vi "Main.vi"(11 "Module Admin":refnum<class "Delacor_lib_QMH_Cloneable Module Admin.lvclass">) -> ()   [LabVIEW 2025, in "Torque Transducer.lvlib"]
doc: "This template is based off of the Queued Message Handler design pattern and the Queued Message Handler project template that ships with LabVIEW.\n\nThe main difference is that the queue is private to this module and communication between modules is performed via Broadcast and Request events.\n\nRequest events are wrapped in public API methods and are handled in the Event Handling Loop (EHL) of this VI. Any module can register for Broadcast events sent by this module. The EHL generates messages based on user interface actions.\n\nThe Message Handling Loop (MHL) processes messages generated by the EHL, or by other messages. The messages are string values, so new messages can be added easily to the Message Cases case structure in the MHL. Each message cluster can also provide an optional value for Message Data, which is a variant that can be converted to whatever message-specific data is required.\n_____\nBased on DQMH Dev Tools: Project Template 7.1.2.1547."
uses:
  Torque Transducer.lvlib
  <vilib>/Delacor/Delacor QMH/Libraries/Cloneable Module Admin_class/Delacor_lib_QMH_Cloneable Module Admin.lvclass
  Module Data--cluster.ctl
  Classes/Torque Transducer/Torque Transducer.lvclass
  <vilib>/Delacor/Delacor QMH/Libraries/Cloneable Module Admin_class/Delacor_lib_QMH_Cloneable Module Admin.lvclass/Delacor_lib_QMH_Cloneable Module Admin.ctl
  <vilib>/Delacor/Delacor QMH/Libraries/Message Queue_class/Delacor_lib_QMH_Message Queue.lvclass/Delacor_lib_QMH_Message Queue.ctl
  Stop Argument--cluster.ctl
  <vilib>/Delacor/Delacor QMH/Libraries/Module Admin_class/Delacor_lib_QMH_Module Admin.lvclass/Delacor_lib_QMH_Module Admin.ctl
  Get Torque DVR Argument--cluster.ctl
  Get Torque DVR (Reply Payload)--cluster.ctl
  read torque Argument--cluster.ctl
  read torque (Reply Payload)--cluster.ctl
  close Argument--cluster.ctl
  close (Reply Payload)--cluster.ctl
  read config Argument--cluster.ctl
  read config (Reply Payload)--cluster.ctl
  init daq Argument--cluster.ctl
  init daq (Reply Payload)--cluster.ctl
  <vilib>/Utility/miscctls.llb/LVPointTypeDef.ctl
  <vilib>/Delacor/Delacor QMH/Libraries/Cloneable Module Admin_class/Delacor_lib_QMH_Get Module ID.vi
  <vilib>/Delacor/Delacor QMH/Libraries/Message Queue_class/Delacor_lib_QMH_Enqueue Message (Single).vi
  <vilib>/Delacor/Delacor QMH/Libraries/Module Admin_class/Delacor_lib_QMH_Get External Launch.vi
  <vilib>/Delacor/Delacor QMH/Libraries/Message Queue_class/Delacor_lib_QMH_Message Queue.lvclass
panel:
  out "Stop the VI":bool
  out "error out":errorcluster
  out "Status":string
  in  "Simulate EHL Error":bool
  in  "Simulate MHL Error":bool
  # "Other processes communicate with this Module via its Public API (wrappers for its Request Events).\n\nThis Module communicates with other processes via its Broadcast Events.\nAny process that wants to receive these messages can register for this module's Broadcast events."
  # "This template is for the DQMH framework. See the block diagram for more information on how to use this template."
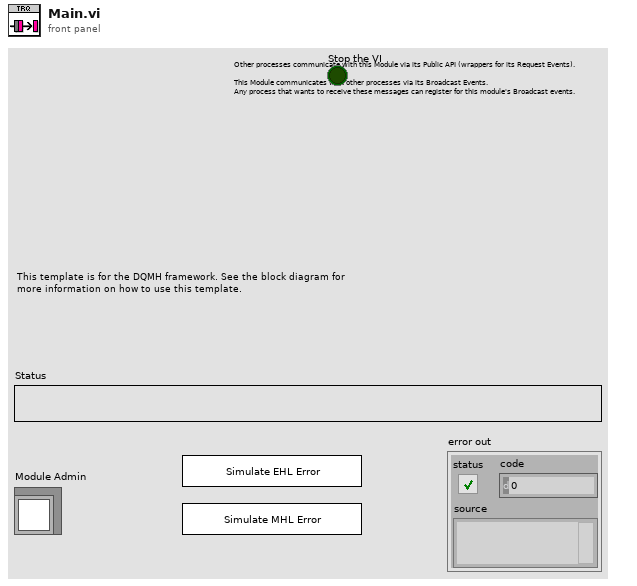
[diagram p1: front panel]
types:
  T1 = typedef "Torque Transducer.lvlib/Request Events--cluster.ctl" = cluster{"Stop Module":refnum<user-event>, "Show Panel":refnum<user-event>, "Hide Panel":refnum<user-event>, "Show Diagram":refnum<user-event>, "Get Module Execution Status":refnum<user-event>, "Get Torque DVR":refnum<user-event>, "read torque":refnum<user-event>, "close":refnum<user-event>, "read config":refnum<user-event>, "init":refnum<user-event>, "init daq":refnum<user-event>}
  T2 = typedef "Torque Transducer.lvlib/Module Data--cluster.ctl" = cluster{"Status":string, "Torque Transducer.lvclass":refnum<class "Torque Transducer.lvclass">}
  T3 = enum32{"invalid lock state", "Not Locked", "Locked (No Password)", "Password-protected"}
  T4 = typedef "Torque Transducer.lvlib/Stop Argument--cluster.ctl" = cluster{"Module ID":i32, "Origin":string, "Exit via Stop Module Req?":bool, "Wait for Module to stop?":bool}
  T5 = typedef "Torque Transducer.lvlib/Get Torque DVR Argument--cluster.ctl" = cluster{"Module ID":i32, "Wait Notifier":refnum<notifier>, "wait for reply":bool}
  T6 = typedef "Torque Transducer.lvlib/read torque Argument--cluster.ctl" = cluster{"Module ID":i32, "Wait Notifier":refnum<notifier>, "wait for reply":bool}
  T7 = typedef "Torque Transducer.lvlib/close Argument--cluster.ctl" = cluster{"Module ID":i32, "Wait Notifier":refnum<notifier>, "wait for reply":bool}
  T8 = typedef "Torque Transducer.lvlib/read config Argument--cluster.ctl" = cluster{"Module ID":i32, "config file path":path, "Wait Notifier":refnum<notifier>, "wait for reply":bool}
  T9 = typedef "Torque Transducer.lvlib/init daq Argument--cluster.ctl" = cluster{"Module ID":i32, "Torque Value":refnum<data-value>, "Wait Notifier":refnum<notifier>, "wait for reply":bool}
  T10 = typedef "LVPointTypeDef.ctl" = cluster{"Horizontal":i16, "Vertical":i16}
  T11 = enum32{"Invalid", "Standard", "Closed", "Hidden", "Minimized", "Maximized"}
  T12 = typedef "Torque Transducer.lvlib/Get Torque DVR (Reply Payload)--cluster.ctl" = cluster{"Module ID":i32, "Numeric":dbl, "Time Stamp":timestamp, "error":errorcluster}
  T13 = typedef "Torque Transducer.lvlib/read torque (Reply Payload)--cluster.ctl" = cluster{"Module ID":i32, "error":errorcluster}
  T14 = typedef "Torque Transducer.lvlib/close (Reply Payload)--cluster.ctl" = cluster{"Module ID":i32, "error":errorcluster}
  T15 = typedef "Torque Transducer.lvlib/read config (Reply Payload)--cluster.ctl" = cluster{"Module ID":i32, "error":errorcluster}
  T16 = typedef "Torque Transducer.lvlib/init daq (Reply Payload)--cluster.ctl" = cluster{"Module ID":i32, "error":errorcluster}
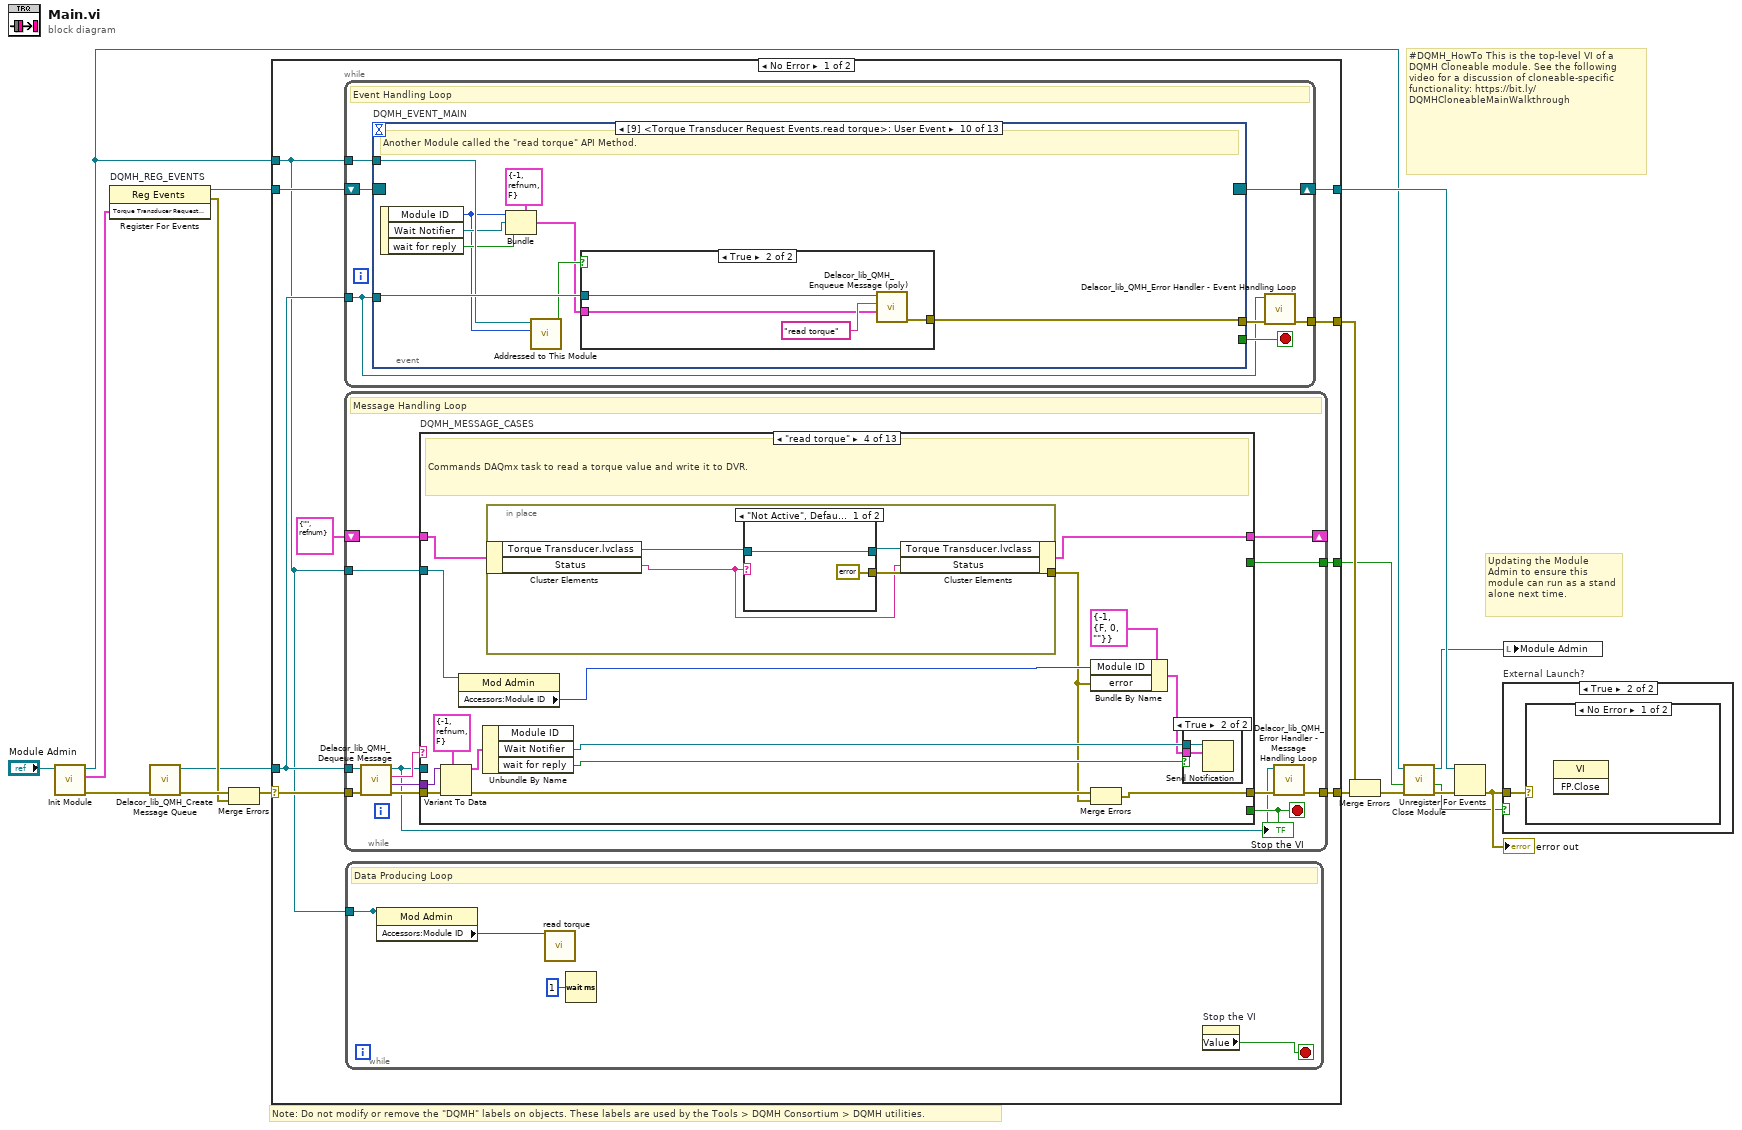
[diagram p0: block diagram]
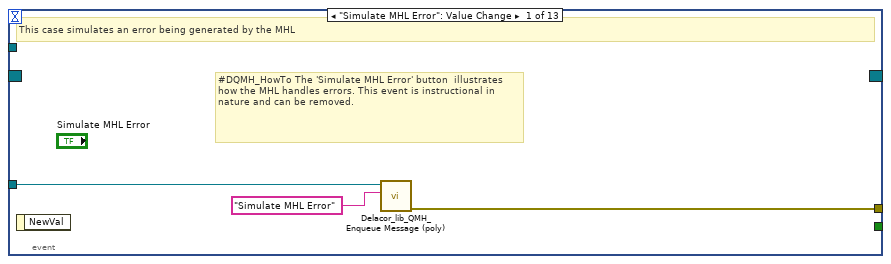
[diagram p2: hidden frame]
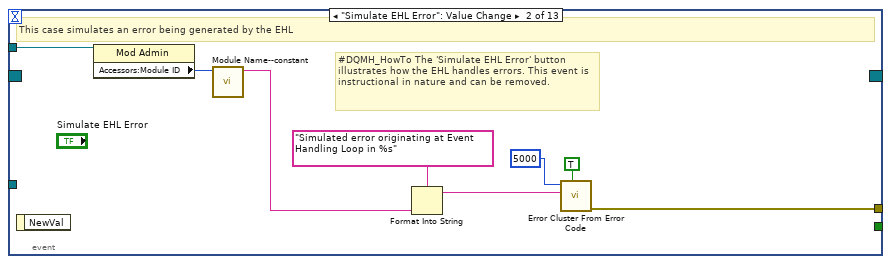
[diagram p3: hidden frame]
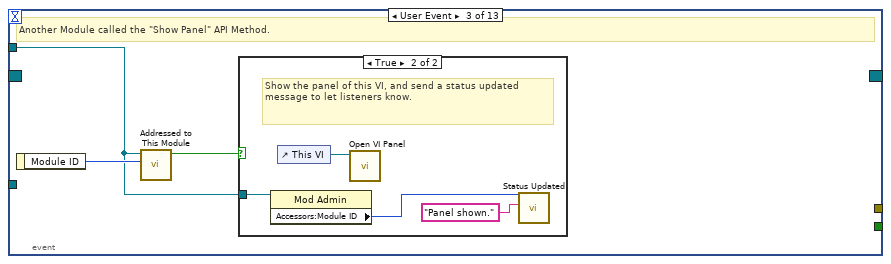
[diagram p4: hidden frame]
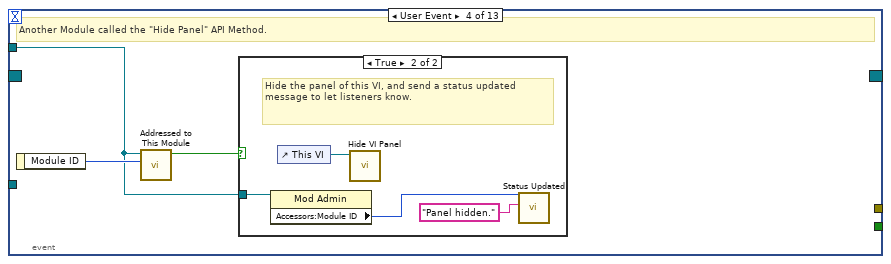
[diagram p6: hidden frame]
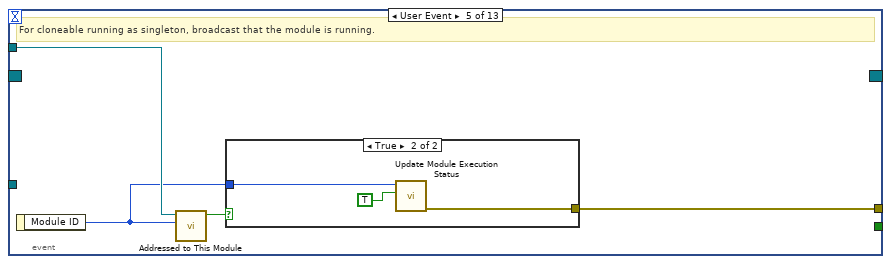
[diagram p8: hidden frame]
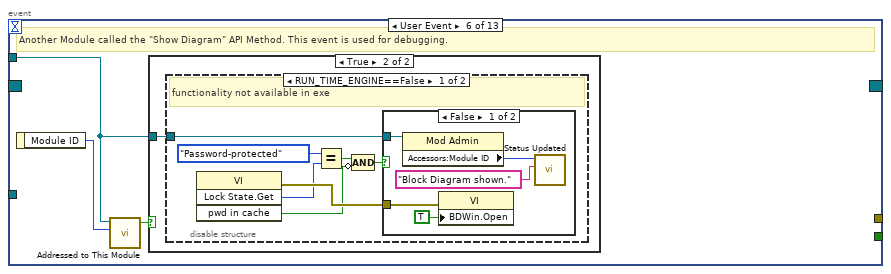
[diagram p10: hidden frame]
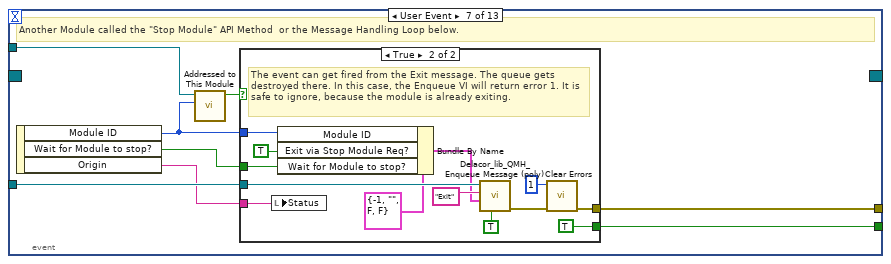
[diagram p14: hidden frame]
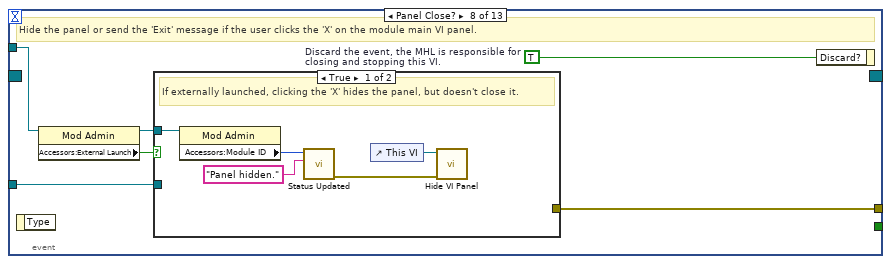
[diagram p16: hidden frame]
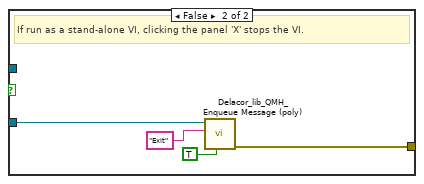
[diagram p17: hidden frame]
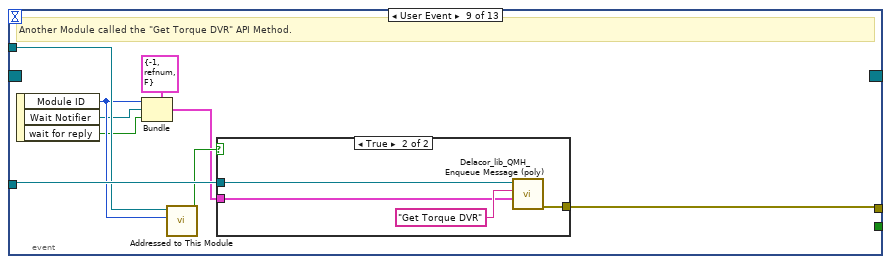
[diagram p18: hidden frame]
diagram:
  # "#DQMH_HowTo This is the top-level VI of a DQMH Cloneable module. See the following video for a discussion of cloneable-specific functionality: https://bit.ly/DQMHCloneableMainWalkthrough"
  # "Note: Do not modify or remove the \"DQMH\" labels on objects. These labels are used by the Tools > DQMH Consortium > DQMH utilities."
  # "Updating the Module Admin to ensure this module can run as a stand alone next time."
  n1 = call "Init Module.vi"("Cloneable Module Admin in"="Module Admin") -> ("error out"=w15:errorcluster, "Torque Transducer Request Events"=w7:T1, "Cloneable Module Admin out"=w4:refnum<class "Delacor_lib_QMH_Cloneable Module Admin.lvclass">)  [unwired: 8 in]
  n2 = register-events "DQMH_REG_EVENTS"(w7) -> (reference out=w8:refnum<event-registration>, error out=w10:errorcluster)  [unwired: 2 in]
  n3 = call <vilib>:"Delacor_lib_QMH_Create Message Queue.vi"("error in"=w15) -> ("error out"=w12:errorcluster, "Message Queue"=w6:refnum<class "Delacor_lib_QMH_Message Queue.lvclass">)  [unwired: 9 in]
  n4 = Merge Errors(w12, w10) -> (w11:errorcluster)
  n5 = case shown="No Error" w11 {
    selector: w11 -> [w25 w416]
    tunnel: [w27 w415] -> w16
    tunnel: [w24 w414] -> w9
    tunnel: w8 -> [w22 w414]
    tunnel: w6 -> [w21 w407]
    tunnel: [w26 _] -> w17
    tunnel: w4 -> [w19 w410]
    tunnel: [w20 _] -> w2
    frame No Error {
      n6 = while {
        tunnel: w21 -> [w32]
        shift-right: [w35] -> w24
        shift-left: w22 -> [w36]
        tunnel: [w37] -> w26
        tunnel: w19 -> [w33]
        stop <- w34 stop-if-true
        # "Event Handling Loop"
        n7 = event "DQMH_EVENT_MAIN" shown="[9] <Torque Transducer Request Events.read torque>: User Event" {
          selector: w36 -> [_ _ _ _ _ _ _ _ _ _ _ _ _]
          dyn-events: [_ _ _ _ _ _ _ _ _ _ _ _ _] -> w35
          timeout: _ -> [_ _ _ _ _ _ _ _ _ _ _ _ _]
          tunnel: [_ _ _ _ _ _ w90 _ _ _ _ _ _] -> w34
          tunnel: w32 -> [w40 _ _ _ _ _ w93 w110 w131 w144 w157 w171 w185]
          tunnel: [w41 w49 _ _ w67 _ w94 w113 w123 w139 w149 w162 w176] -> w38
          tunnel: w33 -> [_ w48 w50 w57 w65 w71 w92 w111 w129 w142 w155 w169 w183]
          event "Simulate MHL Error": Value Change {
            # "#DQMH_HowTo The 'Simulate MHL Error' button  illustrates how the MHL handles errors. This event is instructional in nature and can be removed."
            # "This case simulates an error being generated by the MHL"
            n8 = event-data() -> ()  [unwired: 1 in, 1 out]
            n9 = call-poly <vilib>:"Delacor_lib_QMH_Enqueue Message (poly).vi"("Message"="Simulate MHL Error", "Message Queue in"=w40) -> ("error out"=w41:errorcluster)  [unwired: 8 in, 1 out]
          }
          event "Simulate EHL Error": Value Change {
            # "#DQMH_HowTo The 'Simulate EHL Error' button  illustrates how the EHL handles errors. This event is instructional in nature and can be removed."
            # "This case simulates an error being generated by the EHL"
            n10 = event-data() -> ()  [unwired: 1 in, 1 out]
            n11 = property on="Property Node" class="Mod Admin"(reference=w48) -> ("Accessors:Module ID"=w47:i32)  [unwired: 1 in, 2 out]
            n12 = call "Module Name--constant.vi"("Module ID"=w47) -> ("Module Name"=w42:string)  [unwired: 10 in]
            n13 = Format Into String(format string="Simulated error originating at Event Handling Loop in %s", w42) -> (resulting string=w45:string)  [unwired: 2 in, 1 out]
            n14 = call <vilib>:"Error Cluster From Error Code.vi"("show call chain? (False)"=TRUE, "error message (\"\")"=w45, "error code (0)"=5000) -> ("error out"=w49:errorcluster)  [unwired: 6 in]
          }
          event User Event {
            # "Another Module called the \"Show Panel\" API Method."
            n15 = event-data() -> ("Module ID"=w51:i32)  [unwired: 1 in]
            n16 = call "Addressed to This Module.vi"("Module ID from Argument"=w51, "Module Admin"=w50) -> ("Addressed to this instance?"=w52:bool)  [unwired: 8 in, 1 out]
            n17 = case shown="True" w52 {
              tunnel: w50 -> [_ w54]
              frame False {
              }
              frame True {
                # "Show the panel of this VI, and send a status updated message to let listeners know."
                n18 = property on="Property Node" class="Mod Admin"(reference=w54) -> ("Accessors:Module ID"=w53:i32)  [unwired: 1 in, 2 out]
                n19 = control-ref of="This VI"() -> (w56:refnum<vi>)
                n20 = call "Open VI Panel.vi"("VI"=w56) -> ()  [unwired: 10 in, 1 out]
                n21 = call "Status Updated.vi"("Status"="Panel shown." ("format string"), "Module ID"=w53) -> ()  [unwired: 9 in, 1 out]
              }
            }
          }
          event User Event {
            # "Another Module called the \"Hide Panel\" API Method."
            n22 = event-data() -> ("Module ID"=w58:i32)  [unwired: 1 in]
            n23 = call "Addressed to This Module.vi"("Module ID from Argument"=w58, "Module Admin"=w57) -> ("Addressed to this instance?"=w59:bool)  [unwired: 8 in, 1 out]
            n24 = case shown="True" w59 {
              tunnel: w57 -> [_ w61]
              frame False {
              }
              frame True {
                # "Hide the panel of this VI, and send a status updated message to let listeners know."
                n25 = property on="Property Node" class="Mod Admin"(reference=w61) -> ("Accessors:Module ID"=w60:i32)  [unwired: 1 in, 2 out]
                n26 = control-ref of="This VI"() -> (w63:refnum<vi>)
                n27 = call "Hide VI Panel.vi"("VI"=w63) -> ()  [unwired: 10 in, 1 out]
                n28 = call "Status Updated.vi"("Status"="Panel hidden." ("format string"), "Module ID"=w60) -> ()  [unwired: 9 in, 1 out]
              }
            }
          }
          event User Event {
            # "For cloneable running as singleton, broadcast that the module is running."
            n29 = event-data() -> ("Module ID"=w64:i32)  [unwired: 1 in]
            n30 = call "Addressed to This Module.vi"("Module ID from Argument"=w64, "Module Admin"=w65) -> ("Addressed to this instance?"=w66:bool)  [unwired: 8 in, 1 out]
            n31 = case shown="True" w66 {
              tunnel: [_ w70] -> w67
              tunnel: w64 -> [_ w69]
              frame False {
              }
              frame True {
                n32 = call "Update Module Execution Status.vi"("Running?"=TRUE, "Module ID"=w69) -> ("error out"=w70:errorcluster)  [unwired: 9 in]
              }
            }
          }
          event User Event {
            # "Another Module called the \"Show Diagram\" API Method. This event is used for debugging."
            n33 = event-data() -> ("Module ID"=w72:i32)  [unwired: 1 in]
            n34 = call "Addressed to This Module.vi"("Module ID from Argument"=w72, "Module Admin"=w71) -> ("Addressed to this instance?"=w73:bool)  [unwired: 8 in, 1 out]
            n35 = case shown="True" w73 {
              tunnel: w71 -> [_ w74]
              frame False {
              }
              frame True {
                n36 = disable-structure shown="RUN_TIME_ENGINE==False" {
                  disable-tunnel: w74 -> [w75 _]
                  frame condition #0 (active) {
                    # "functionality not available in exe"
                    n37 = invoke on="Invoke Node" class="VI" method="Lock State.Get"() -> (error out=w81:errorcluster, "Get Lock State"=w80:T3, "pwd in cache"=w77:bool)  [unwired: 4 in, 1 out]
                    n38 = Equal?(x=T3."Password-protected", y=w80) -> (x = y?=w78:bool)
                    n39 = Compound Arithmetic op=AND(w78, invert w77) -> (w76:bool)
                    n40 = case shown="False" w76 {
                      tunnel: w81 -> [w86 _]
                      tunnel: w75 -> [w83 _]
                      frame False {
                        n41 = property on="Property Node" class="Mod Admin"(reference=w83) -> ("Accessors:Module ID"=w82:i32)  [unwired: 1 in, 2 out]
                        n42 = property on="Property Node" class="VI"(error in=w86, "BDWin.Open"=TRUE ("Block Diagram Window:Open")) -> ()  [unwired: 1 in, 2 out]
                        n43 = call "Status Updated.vi"("Status"="Block Diagram shown." ("format string"), "Module ID"=w82) -> ()  [unwired: 9 in, 1 out]
                      }
                      frame True {
                        # "Password-protected VI, and the password is not in the cache. Do not show the diagram."
                      }
                    }
                  }
                  frame condition #1 {
                  }
                }
              }
            }
          }
          event User Event {
            # "Another Module called the \"Stop Module\" API Method  or the Message Handling Loop below."
            n44 = event-data() -> ("Module ID"=w88:i32, "Wait for Module to stop?"=w89:bool, "Origin"=w87:string)  [unwired: 1 in]
            n45 = call "Addressed to This Module.vi"("Module ID from Argument"=w88, "Module Admin"=w92) -> ("Addressed to this instance?"=w91:bool)  [unwired: 8 in, 1 out]
            n46 = case shown="True" w91 {
              tunnel: [_ w106] -> w94
              tunnel: w93 -> [_ w102]
              tunnel: [_ TRUE] -> w90
              tunnel: w89 -> [_ w97]
              tunnel: w88 -> [_ w99]
              tunnel: w87 -> [_ w95]
              frame False {
              }
              frame True {
                # "The event can get fired from the Exit message. The queue gets destroyed there. In this case, the Enqueue VI will return error 1. It is safe to ignore, because the module is already exiting."
                n47 = local write "Status"(w95) -> ()
                n48 = Bundle By Name(cluster=T4 {"Module ID"=-1, "Origin"="", "Exit via Stop Module Req?"=FALSE, "Wait for Module to stop?"=FALSE} ("Stop Argument"), "Module ID"=w99, "Exit via Stop Module Req?"=TRUE, "Wait for Module to stop?"=w97) -> (w96:T4)
                n49 = call-poly <vilib>:"Delacor_lib_QMH_Enqueue Message (poly).vi"("Priority Message? (F)"=TRUE, "Message Data"=w96, "Message"="Exit", "Message Queue in"=w102) -> ("error out"=w107:errorcluster)  [unwired: 6 in, 1 out]
                n50 = call <vilib>:"Clear Errors.vi"("error in (no error)"=w107, "specific error code to clear (0: all)"=1) -> ("error out"=w106:errorcluster)  [unwired: 4 in, 1 out]
              }
            }
          }
          event Panel Close? {
            w112 = TRUE  # Discard the event, the MHL is responsible for closing and stopping this VI.
            # "Hide the panel or send the 'Exit' message if the user clicks the 'X' on the module main VI panel."
            n51 = event-data() -> ()  [unwired: 1 in, 1 out]
            n52 = property on="Property Node" class="Mod Admin"(reference=w111) -> (reference out=w108:refnum<class "Delacor_lib_QMH_Cloneable Module Admin.lvclass">, "Accessors:External Launch"=w109:bool)  [unwired: 1 in, 1 out]
            n53 = case shown="True" w109 {
              tunnel: w110 -> [_ w121]
              tunnel: [_ w122] -> w113
              tunnel: w108 -> [w116 _]
              frame True {
                # "If externally launched, clicking the 'X' hides the panel, but doesn't close it."
                n54 = property on="Property Node" class="Mod Admin"(reference=w116) -> ("Accessors:Module ID"=w115:i32)  [unwired: 1 in, 2 out]
                n55 = call "Status Updated.vi"("Status"="Panel hidden." ("format string"), "Module ID"=w115) -> ("error out"=w114:errorcluster)  [unwired: 9 in]
                n56 = control-ref of="This VI"() -> (w118:refnum<vi>)
                n57 = call "Hide VI Panel.vi"("error in"=w114, "VI"=w118) -> ()  [unwired: 9 in, 1 out]
              }
              frame False {
                # "If run as a stand-alone VI, clicking the panel 'X' stops the VI."
                n58 = call-poly <vilib>:"Delacor_lib_QMH_Enqueue Message (poly).vi"("Priority Message? (F)"=TRUE, "Message"="Exit", "Message Queue in"=w121) -> ("error out"=w122:errorcluster)  [unwired: 7 in, 1 out]
              }
            }
            n59 = event-data ("Event Filter Node")("Discard?"=w112) -> ()  [unwired: 1 in, 1 out]
          }
          event User Event {
            # "Another Module called the \"Get Torque DVR\" API Method."
            n60 = event-data() -> ("Module ID"=w126:i32, "Wait Notifier"=w125:refnum<notifier>, "wait for reply"=w124:bool)  [unwired: 1 in]
            n61 = Bundle(cluster=T5 {"Module ID"=-1, "Wait Notifier"=refnum, "wait for reply"=FALSE} ("Get Torque DVR Argument"), "Module ID"=w126, "Wait Notifier"=w125, "wait for reply"=w124) -> (w127:T5)
            n62 = call "Addressed to This Module.vi"("Module ID from Argument"=w126, "Module Admin"=w129) -> ("Addressed to this instance?"=w130:bool)  [unwired: 8 in, 1 out]
            n63 = case shown="True" w130 {
              tunnel: w131 -> [_ w135]
              tunnel: w127 -> [_ w133]
              tunnel: [_ w132] -> w123
              frame False {
              }
              frame True {
                n64 = call-poly <vilib>:"Delacor_lib_QMH_Enqueue Message (poly).vi"("Message Data"=w133, "Message"="Get Torque DVR", "Message Queue in"=w135) -> ("error out"=w132:errorcluster)  [unwired: 7 in, 1 out]
              }
            }
          }
          event User Event {
            # "Another Module called the \"read torque\" API Method."
            n65 = event-data() -> ("Module ID"=w136:i32, "Wait Notifier"=w138:refnum<notifier>, "wait for reply"=w137:bool)  [unwired: 1 in]
            n66 = Bundle(cluster=T6 {"Module ID"=-1, "Wait Notifier"=refnum, "wait for reply"=FALSE} ("read torque Argument"), "Module ID"=w136, "Wait Notifier"=w138, "wait for reply"=w137) -> (w140:T6)
            n67 = call "Addressed to This Module.vi"("Module ID from Argument"=w136, "Module Admin"=w142) -> ("Addressed to this instance?"=w143:bool)  [unwired: 8 in, 1 out]
            n68 = case shown="True" w143 {
              tunnel: w144 -> [_ w148]
              tunnel: w140 -> [_ w146]
              tunnel: [_ w145] -> w139
              frame False {
              }
              frame True {
                n69 = call-poly <vilib>:"Delacor_lib_QMH_Enqueue Message (poly).vi"("Message Data"=w146, "Message"="read torque", "Message Queue in"=w148) -> ("error out"=w145:errorcluster)  [unwired: 7 in, 1 out]
              }
            }
          }
          event User Event {
            # "Another Module called the \"close\" API Method."
            n70 = event-data() -> ("Module ID"=w152:i32, "Wait Notifier"=w151:refnum<notifier>, "wait for reply"=w150:bool)  [unwired: 1 in]
            n71 = Bundle(cluster=T7 {"Module ID"=-1, "Wait Notifier"=refnum, "wait for reply"=FALSE} ("close Argument"), "Module ID"=w152, "Wait Notifier"=w151, "wait for reply"=w150) -> (w153:T7)
            n72 = call "Addressed to This Module.vi"("Module ID from Argument"=w152, "Module Admin"=w155) -> ("Addressed to this instance?"=w156:bool)  [unwired: 8 in, 1 out]
            n73 = case shown="True" w156 {
              tunnel: w157 -> [_ w161]
              tunnel: w153 -> [_ w159]
              tunnel: [_ w158] -> w149
              frame False {
              }
              frame True {
                n74 = call-poly <vilib>:"Delacor_lib_QMH_Enqueue Message (poly).vi"("Message Data"=w159, "Message"="close", "Message Queue in"=w161) -> ("error out"=w158:errorcluster)  [unwired: 7 in, 1 out]
              }
            }
          }
          event User Event {
            # "Another Module called the \"read config\" API Method."
            n75 = event-data() -> ("Module ID"=w166:i32, "config file path"=w165:path, "Wait Notifier"=w164:refnum<notifier>, "wait for reply"=w163:bool)  [unwired: 1 in]
            n76 = Bundle(cluster=T8 {"Module ID"=-1, "config file path"=path "", "Wait Notifier"=refnum, "wait for reply"=FALSE} ("read config Argument"), "Module ID"=w166, "config file path"=w165, "Wait Notifier"=w164, "wait for reply"=w163) -> (w167:T8)
            n77 = call "Addressed to This Module.vi"("Module ID from Argument"=w166, "Module Admin"=w169) -> ("Addressed to this instance?"=w170:bool)  [unwired: 8 in, 1 out]
            n78 = case shown="True" w170 {
              tunnel: w171 -> [_ w175]
              tunnel: w167 -> [_ w173]
              tunnel: [_ w172] -> w162
              frame False {
              }
              frame True {
                n79 = call-poly <vilib>:"Delacor_lib_QMH_Enqueue Message (poly).vi"("Message Data"=w173, "Message"="read config", "Message Queue in"=w175) -> ("error out"=w172:errorcluster)  [unwired: 7 in, 1 out]
              }
            }
          }
          event User Event {
            # "Another Module called the \"init daq\" API Method."
            n80 = event-data() -> ("Module ID"=w180:i32, "Torque Value"=w179:refnum<data-value>, "Wait Notifier"=w178:refnum<notifier>, "wait for reply"=w177:bool)  [unwired: 1 in]
            n81 = Bundle(cluster=T9 {"Module ID"=-1, "Torque Value"=refnum, "Wait Notifier"=refnum, "wait for reply"=FALSE} ("init daq Argument"), "Module ID"=w180, "Torque Value"=w179, "Wait Notifier"=w178, "wait for reply"=w177) -> (w181:T9)
            n82 = call "Addressed to This Module.vi"("Module ID from Argument"=w180, "Module Admin"=w183) -> ("Addressed to this instance?"=w184:bool)  [unwired: 8 in, 1 out]
            n83 = case shown="True" w184 {
              tunnel: w185 -> [_ w189]
              tunnel: w181 -> [_ w187]
              tunnel: [_ w186] -> w176
              frame False {
              }
              frame True {
                n84 = call-poly <vilib>:"Delacor_lib_QMH_Enqueue Message (poly).vi"("Message Data"=w187, "Message"="init daq", "Message Queue in"=w189) -> ("error out"=w186:errorcluster)  [unwired: 7 in, 1 out]
              }
            }
          }
        }
        n85 = call-dynamic "Delacor_lib_QMH_Error Handler - Event Handling Loop.vi"("error in"=w38, "Message Queue in"=w32) -> ("dup error in"=w37:errorcluster)  [unwired: 8 in, 1 out]
      }
      n86 = while {
        tunnel: w21 -> [w190]
        shift-right: [w197] -> _
        shift-left: T2 {"Status"="", "Torque Transducer.lvclass"=refnum} ("Data Cluster") -> [w198]
        tunnel: w25 -> [w201]
        tunnel: [w199] -> w27
        tunnel: w19 -> [w192]
        tunnel: [w191] -> w20
        stop <- w196 stop-if-true
        # "Message Handling Loop"
        n87 = call-dynamic "Delacor_lib_QMH_Dequeue Message.vi"("error in"=w201, "Message Queue in"=w190) -> ("error out"=w200:errorcluster, "Message Data"=w194:variant, "Message"=w195:string, "Message Queue out"=w193:refnum<class "Delacor_lib_QMH_Message Queue.lvclass">)  [unwired: 6 in]
        n88 = case "DQMH_MESSAGE_CASES" shown="\"read torque\"" w195 {
          selector: w195 -> [_ _ _ _ _ _ _ _ _ _ _ _ w396]
          tunnel: w193 -> [_ _ _ _ _ _ _ _ _ w351 _ w388 _]
          tunnel: w200 -> [w221 w225 w242 w264 w290 w312 w334 w346 w348 w360 w377 w394 w405]
          tunnel: [w219 w225 w233 w255 w281 w303 w325 w345 w348 w356 w376 w389 w406] -> w202
          tunnel: w198 -> [w212 w224 w230 w252 w278 w300 w322 w344 w347 w355 w374 w387 w403]
          tunnel: [w211 w224 w229 w251 w277 w299 w319 w344 w347 w355 w374 w387 w403] -> w197
          tunnel: [_ _ _ _ _ _ _ _ _ _ _ w386 _] -> w196
          tunnel: w194 -> [_ _ w240 w262 w288 w310 w332 _ _ w354 _ w384 _]
          tunnel: w192 -> [w207 _ w231 w253 w279 w301 w323 _ _ w353 w372 w379 w402]
          tunnel: [_ _ _ _ _ _ _ _ _ _ _ w382 _] -> w191
          frame "Initialize" {
            w204 = "Initial Message" ("Initial Message")
            # "#DQMH_CodeNeeded - Initialize the appearance of the front panel."
            # "#DQMH_CodeNeeded - Initialize your state data here."
            # "Initialize - Any operation that needs to be done before the module can receive messages. Synchronize Caller Events.vi will inform Start Module.vi that the module has launched and is ready to receive messages. Module Did Init.vi will broadcast that the module initialized."
            n89 = call "Synchronize Caller Events.vi"("error in"=w221, "Module Admin"=w207) -> ("error out"=w220:errorcluster, "Module Admin out"=w206:refnum<class "Delacor_lib_QMH_Cloneable Module Admin.lvclass">)  [unwired: 8 in]
            n90 = property on="Property Node" class="Mod Admin"(reference=w206) -> ("Accessors:Module ID"=w203:i32, "Accessors:External Launch"=w208:bool)  [unwired: 1 in, 2 out]
            n91 = call "Module Name--constant.vi"("Module ID"=w203) -> ("Module Name"=w216:string)  [unwired: 10 in]
            n92 = property on="Property Node" class="VI"("Front Panel.Title"=w216) -> (reference out=w218:refnum<vi>, error out=w223:errorcluster)  [unwired: 2 in]
            n93 = Select(t=T11."Hidden" ("State"), s=w208, f=T11."Standard" ("State")) -> (s? t:f=w213:T11)
            n94 = invoke on="Invoke Node" class="VI" method="FP.Open"(reference=w218, error in=w223, "State"=w213) -> (reference out=w217:refnum<vi>, error out=w222:errorcluster)  [unwired: 2 in, 3 out]
            n95 = Bundle By Name(cluster=w212, "Status"=w204) -> (w211:T2)
            n96 = invoke on="Invoke Node" class="VI" method="FP.Center"(reference=w217, error in=w222) -> ()  [unwired: 1 in, 3 out]
            n97 = property on="Pane" class="Pane"("Origin"=T10 {"Horizontal"=0, "Vertical"=0}) -> ()  [unwired: 2 in, 2 out]
            n98 = call "Module Name--constant.vi"("Module ID"=w203) -> ("Module Name"=w209:string)  [unwired: 10 in]
            n99 = call "Module Did Init.vi"("error in"=w220, "Initialized?"=TRUE, "Origin"=w209, "Module ID"=w203) -> ("error out"=w219:errorcluster)  [unwired: 7 in]
            "Status" <- w204
          }
          frame "---Module Specific---" {
            # "Separator -- The following cases handle messages specific to this Module."
          }
          frame "Get Torque DVR" {
            # "Read Torque DVR"
            n100 = Variant To Data(error in=w242, type=T5 {"Module ID"=-1, "Wait Notifier"=refnum, "wait for reply"=FALSE} ("Get Torque DVR Argument"), Variant=w240) -> (data=w238:T5, error out=w241:errorcluster)
            n101 = property class="Mod Admin"(reference=w231) -> ("Accessors:Module ID"=w232:i32)  [unwired: 1 in, 2 out]
            n102 = in-place {
              in-place-border: [w245] -> w228
              in-place-border: [w244] -> w227
              in-place-border: [w243] -> w226
              n103 = in-place-cluster #1(w230) -> ("Torque Transducer.lvclass"=w247:refnum<class "Torque Transducer.lvclass">)
              n104 = call-dynamic "read torque dvr.vi"("Torque Transducer in"=w247) -> ("error out"=w243:errorcluster, "Torque"=w245:dbl, "Time"=w244:timestamp, "Torque Transducer out"=w246:refnum<class "Torque Transducer.lvclass">)  [unwired: 7 in]
              n105 = in-place-cluster #1("Torque Transducer.lvclass"=w246) -> (w229:T2)
            }
            n106 = Unbundle By Name(w238) -> ("Wait Notifier"=w237:refnum<notifier>, "wait for reply"=w236:bool)  [unwired: 1 out]
            n107 = Bundle By Name(cluster=T12 {"Module ID"=-1, "Numeric"=0.0, "Time Stamp"=timestamp(0 s since 1904-01-01), "error"={"status"=FALSE, "code"=0, "source"=""}} ("Get Torque DVR (Reply Payload)"), "Module ID"=w232, "Numeric"=w228, "Time Stamp"=w227, "error"=w226) -> (w235:T12)
            n108 = Merge Errors(w241, w226) -> (w233:errorcluster)
            n109 = case "DQMH_FIRE_NOTIFIER" shown="True" w236 {
              tunnel: w237 -> [_ w249]
              tunnel: w235 -> [_ w248]
              frame False {
              }
              frame True {
                n110 = Send Notification(notification=w248, notifier=w249) -> ()  [unwired: 1 in, 2 out]
              }
            }
          }
          frame "read torque" {
            # "Commands DAQmx task to read a torque value and write it to DVR."
            n111 = Variant To Data(error in=w264, type=T6 {"Module ID"=-1, "Wait Notifier"=refnum, "wait for reply"=FALSE} ("read torque Argument"), Variant=w262) -> (data=w260:T6, error out=w263:errorcluster)
            n112 = property class="Mod Admin"(reference=w253) -> ("Accessors:Module ID"=w254:i32)  [unwired: 1 in, 2 out]
            n113 = Unbundle By Name(w260) -> ("Wait Notifier"=w259:refnum<notifier>, "wait for reply"=w258:bool)  [unwired: 1 out]
            n114 = in-place {
              in-place-border: [w266] -> w250
              n115 = in-place-cluster #2(w252) -> ("Torque Transducer.lvclass"=w268:refnum<class "Torque Transducer.lvclass">, "Status"=w265:string)
              n116 = case shown="\"Not Active\", Default" w265 {
                tunnel: w268 -> [w270 w273]
                tunnel: [w270 w272] -> w267
                tunnel: [errorcluster {"status"=FALSE, "code"=0, "source"=""} ("error out") w271] -> w266
                frame "Not Active", Default {
                }
                frame "Active" {
                  n117 = call-dynamic "read torque.vi"("Torque Transducer in"=w273) -> ("error out"=w271:errorcluster, "Torque Transducer out"=w272:refnum<class "Torque Transducer.lvclass">)  [unwired: 9 in]
                }
              }
              n118 = in-place-cluster #2("Torque Transducer.lvclass"=w267, "Status"=w265) -> (w251:T2)
            }
            n119 = Bundle By Name(cluster=T13 {"Module ID"=-1, "error"={"status"=FALSE, "code"=0, "source"=""}} ("read torque (Reply Payload)"), "Module ID"=w254, "error"=w250) -> (w257:T13)
            n120 = Merge Errors(w263, w250) -> (w255:errorcluster)
            n121 = case "DQMH_FIRE_NOTIFIER" shown="True" w258 {
              tunnel: w259 -> [_ w275]
              tunnel: w257 -> [_ w274]
              frame False {
              }
              frame True {
                n122 = Send Notification(notification=w274, notifier=w275) -> ()  [unwired: 1 in, 2 out]
              }
            }
          }
          frame "close" {
            # "Close DAQmx task"
            n123 = Variant To Data(error in=w290, type=T7 {"Module ID"=-1, "Wait Notifier"=refnum, "wait for reply"=FALSE} ("close Argument"), Variant=w288) -> (data=w286:T7, error out=w289:errorcluster)
            n124 = property class="Mod Admin"(reference=w279) -> ("Accessors:Module ID"=w280:i32)  [unwired: 1 in, 2 out]
            n125 = Unbundle By Name(w286) -> ("Wait Notifier"=w285:refnum<notifier>, "wait for reply"=w284:bool)  [unwired: 1 out]
            n126 = in-place {
              in-place-border: [w292] -> w276
              n127 = in-place-cluster #3(w278) -> ("Torque Transducer.lvclass"=w294:refnum<class "Torque Transducer.lvclass">)  [unwired: 1 out]
              n128 = call-dynamic "close.vi"("Torque Transducer in"=w294) -> ("error out"=w292:errorcluster, "Torque Transducer out"=w293:refnum<class "Torque Transducer.lvclass">)  [unwired: 9 in]
              n129 = in-place-cluster #3("Torque Transducer.lvclass"=w293, "Status"="Not Active") -> (w277:T2)
            }
            n130 = Bundle By Name(cluster=T14 {"Module ID"=-1, "error"={"status"=FALSE, "code"=0, "source"=""}} ("close (Reply Payload)"), "Module ID"=w280, "error"=w276) -> (w283:T14)
            n131 = Merge Errors(w289, w276) -> (w281:errorcluster)
            n132 = case "DQMH_FIRE_NOTIFIER" shown="True" w284 {
              tunnel: w285 -> [_ w296]
              tunnel: w283 -> [_ w295]
              frame False {
              }
              frame True {
                n133 = Send Notification(notification=w295, notifier=w296) -> ()  [unwired: 1 in, 2 out]
              }
            }
          }
          frame "read config" {
            # "Reads important Channel names and settings from .json config file"
            n134 = property class="Mod Admin"(reference=w301) -> ("Accessors:Module ID"=w302:i32)  [unwired: 1 in, 2 out]
            n135 = Variant To Data(error in=w312, type=T8 {"Module ID"=-1, "config file path"=path "", "Wait Notifier"=refnum, "wait for reply"=FALSE} ("read config Argument"), Variant=w310) -> (data=w308:T8, error out=w311:errorcluster)
            n136 = Unbundle By Name(w308) -> ("config file path"=w297:path, "Wait Notifier"=w307:refnum<notifier>, "wait for reply"=w306:bool)  [unwired: 1 out]
            n137 = in-place {
              in-place-border: [w314] -> w298
              in-place-border: w297 -> [w313]
              n138 = in-place-cluster #4(w300) -> ("Torque Transducer.lvclass"=w316:refnum<class "Torque Transducer.lvclass">)
              n139 = call-dynamic "read config.vi"("Path"=w313, "Torque Transducer in"=w316) -> ("error out"=w314:errorcluster, "Torque Transducer out"=w315:refnum<class "Torque Transducer.lvclass">)  [unwired: 8 in]
              n140 = in-place-cluster #4("Torque Transducer.lvclass"=w315) -> (w299:T2)
            }
            n141 = Bundle By Name(cluster=T15 {"Module ID"=-1, "error"={"status"=FALSE, "code"=0, "source"=""}} ("read config (Reply Payload)"), "Module ID"=w302, "error"=w298) -> (w305:T15)
            n142 = Merge Errors(w311, w298) -> (w303:errorcluster)
            n143 = case "DQMH_FIRE_NOTIFIER" shown="True" w306 {
              tunnel: w307 -> [_ w318]
              tunnel: w305 -> [_ w317]
              frame False {
              }
              frame True {
                n144 = Send Notification(notification=w317, notifier=w318) -> ()  [unwired: 1 in, 2 out]
              }
            }
          }
          frame "init daq" {
            # "Initialize DAQmx channel & DVR."
            n145 = Variant To Data(error in=w334, type=T9 {"Module ID"=-1, "Torque Value"=refnum, "Wait Notifier"=refnum, "wait for reply"=FALSE} ("init daq Argument"), Variant=w332) -> (data=w330:T9, error out=w333:errorcluster)
            n146 = property class="Mod Admin"(reference=w323) -> ("Accessors:Module ID"=w324:i32)  [unwired: 1 in, 2 out]
            n147 = Unbundle By Name(w330) -> ("Torque Value"=w321:refnum<data-value>, "Wait Notifier"=w329:refnum<notifier>, "wait for reply"=w328:bool)  [unwired: 1 out]
            n148 = in-place {
              in-place-border: w321 -> [w337]
              in-place-border: [w336] -> w320
              n149 = in-place-cluster #5(w322) -> ("Torque Transducer.lvclass"=w338:refnum<class "Torque Transducer.lvclass">)  [unwired: 1 out]
              n150 = call-dynamic "init.vi"("Torque Value"=w337, "Torque Transducer in"=w338) -> ("error out"=w336:errorcluster, "Torque Transducer out"=w339:refnum<class "Torque Transducer.lvclass">)  [unwired: 8 in]
              n151 = case shown="No Error" w336 {
                tunnel: ["Active" "Not Active"] -> w335
                frame No Error {
                }
                frame Error {
                }
              }
              n152 = in-place-cluster #5("Torque Transducer.lvclass"=w339, "Status"=w335) -> (w319:T2)
            }
            n153 = Bundle By Name(cluster=T16 {"Module ID"=-1, "error"={"status"=FALSE, "code"=0, "source"=""}} ("init daq (Reply Payload)"), "Module ID"=w324, "error"=w320) -> (w327:T16)
            n154 = Merge Errors(w333, w320) -> (w325:errorcluster)
            n155 = case "DQMH_FIRE_NOTIFIER" shown="True" w328 {
              tunnel: w329 -> [_ w343]
              tunnel: w327 -> [_ w342]
              frame False {
              }
              frame True {
                n156 = Send Notification(notification=w342, notifier=w343) -> ()  [unwired: 1 in, 2 out]
              }
            }
          }
          frame "---Copy This Frame---" {
            # "Duplicate this frame when creating new messages.  Change this comment in the duplicated frame to describe this message."
            n157 = Merge Errors(w346) -> (w345:errorcluster)
          }
          frame "---Exit and Error Handling---" {
            # "Separator - the following cases handle errors and exit messages."
          }
          frame "Error" {
            # "#DQMH_CodeRecommended - If the module is running in standalone mode (External Launch = FALSE), this code will pop up an error dialog and call the 'Exit' message if an error occurs. Add more fine-grained error management here."
            # "Error - Check the error message data and respond accordingly. This message is sent by the \"Error Handler\" VIs at the end of each loop in this application."
            n158 = property on="Property Node" class="Mod Admin"(reference=w353) -> ("Accessors:External Launch"=w352:bool, "Accessors:Module ID"=w350:i32)  [unwired: 1 in, 2 out]
            n159 = Variant To Data(error in=w360, type=errorcluster {"status"=FALSE, "code"=0, "source"=""} ("error constant"), Variant=w354) -> (data=w349:errorcluster, error out=w358:errorcluster)
            n160 = local write "error out"(w349) -> ()
            n161 = call "Error Reported.vi"("Error"=w349, "Module ID"=w350) -> ()  [unwired: 9 in, 1 out]
            n162 = case shown="False" w352 {
              tunnel: [w365 _] -> w357
              tunnel: w351 -> [w363 _]
              tunnel: w349 -> [w364 _]
              frame False {
                n163 = disable-structure shown="Default" {
                  disable-tunnel: w364 -> [w366 _]
                  frame condition #0 (active) {
                    # "If the module is running standalone, then pop up an error dialog and call the \"Exit\" message."
                    n164 = call <vilib>:"Simple Error Handler.vi"("error in (no error)"=w366) -> ()  [unwired: 4 in, 5 out]
                  }
                  frame condition #1 {
                    # "To prevent the Simple Error Handler VI from being loaded (e.g. when deploying to a Real-Time target), add the Conditional Disable Symbol \"DQMH_Disable_SEH\" to your project and set it to TRUE."
                  }
                }
                n165 = call-poly <vilib>:"Delacor_lib_QMH_Enqueue Message (poly).vi"("Priority Message? (F)"=TRUE, "Message"="Exit", "Message Queue in"=w363) -> ("error out"=w365:errorcluster)  [unwired: 7 in, 1 out]
              }
              frame True {
                # "If the module was launched externally, calling the Error Reported broadcast VI is the only action performed by the \"Error\" message. The module's caller can then process the error appropriately."
              }
            }
            n166 = Merge Errors(w358, w357) -> (w356:errorcluster)
          }
          frame "Simulate MHL Error" {
            # "#DQMH_HowTo The 'Simulate MHL Error' button  illustrates how the MHL handles errors. This event is instructional in nature and can be removed."
            # "Simulate an error occurring at the MHL"
            n167 = property on="Property Node" class="Mod Admin"(reference=w372) -> ("Accessors:Module ID"=w373:i32)  [unwired: 1 in, 2 out]
            n168 = call "Module Name--constant.vi"("Module ID"=w373) -> ("Module Name"=w368:string)  [unwired: 10 in]
            n169 = Format Into String(format string="Simulated error originating at Message Handling Loop in %s", w368) -> (resulting string=w369:string)  [unwired: 2 in, 1 out]
            n170 = call <vilib>:"Error Cluster From Error Code.vi"("show call chain? (False)"=TRUE, "error message (\"\")"=w369, "error code (0)"=5001) -> ("error out"=w375:errorcluster)  [unwired: 6 in]
            n171 = Merge Errors(w377, w375) -> (w376:errorcluster)
          }
          frame "Exit" {
            w385 = 91  # 91: not all Exit messages will have an argument
            w386 = TRUE  # Stop the VI
            # "Release the message queue reference"
            # "#DQMH_CodeNeeded - Add any required cleanup code here."
            # "Exit - Exit the application."
            n172 = Variant To Data(error in=w394, type=T4 {"Module ID"=-1, "Origin"="", "Exit via Stop Module Req?"=FALSE, "Wait for Module to stop?"=FALSE} ("Stop Argument"), Variant=w384) -> (data=w381:T4, error out=w390:errorcluster)
            n173 = call <vilib>:"Clear Errors.vi"("error in (no error)"=w390, "specific error code to clear (0: all)"=w385) -> ("error out"=w393:errorcluster)  [unwired: 4 in, 1 out]
            n174 = property on="Property Node" class="Mod Admin"(reference=w379) -> ("Accessors:Module ID"=w378:i32)  [unwired: 1 in, 2 out]
            n175 = control-ref of="This VI"() -> (w380:refnum<vi>)
            n176 = call-dynamic "Delacor_lib_QMH_Release Message Queue.vi"("error in"=w393, "Message Queue"=w388) -> ("error out"=w392:errorcluster)  [unwired: 9 in]
            n177 = call "Handle Exit.vi"("Stop Argument"=w381, "Module Admin in"=w379, "VI reference"=w380) -> ("error out"=w391:errorcluster, "Wait for Stop?"=w382:bool)  [unwired: 7 in]
            n178 = Merge Errors(w392, w391) -> (w389:errorcluster)
            n179 = call "Error Reported.vi"("Error"=w389, "Module ID"=w378) -> ()  [unwired: 9 in, 1 out]
          }
          frame Default {
            # "'Default' case only runs if there is a message that isn't defined in any of the other cases.  Output a programming error."
            n180 = property on="Property Node" class="Mod Admin"(reference=w402) -> ("Accessors:Module ID"=w401:i32)  [unwired: 1 in, 2 out]
            n181 = call "Module Name--constant.vi"("Module ID"=w401) -> ("Module Name"=w395:string)  [unwired: 10 in]
            n182 = Format Into String(format string="The invalid message string \"%s\" was received in the Message Handling Loop for module \"%s\".", w396, w395) -> (resulting string=w398:string)  [unwired: 2 in, 1 out]
            n183 = call <vilib>:"Error Cluster From Error Code.vi"("show call chain? (False)"=TRUE, "error message (\"\")"=w398, "error code (0)"=1) -> ("error out"=w404:errorcluster)  [unwired: 6 in]
            n184 = Merge Errors(w405, w404) -> (w406:errorcluster)
          }
        }
        "Stop the VI" <- w196
        n185 = call-dynamic "Delacor_lib_QMH_Error Handler - Message Handling Loop.vi"("error in"=w202, "Message Queue in"=w193) -> ("dup error in"=w199:errorcluster)  [unwired: 8 in, 1 out]
      }
      n186 = while {
        tunnel: [w30] -> _
        tunnel: w19 -> [w30]
        stop <- w31 stop-if-true
        # "Data Producing Loop"
        n187 = property class="Mod Admin"(reference=w30) -> ("Accessors:Module ID"=w28:i32)  [unwired: 1 in, 2 out]
        n188 = call "read torque.vi"("Module ID"=w28) -> ()  [unwired: 9 in, 2 out]
        n189 = Wait (ms)(milliseconds to wait=u32 1) -> ()  [unwired: 1 out]
        n190 = property on="Stop the VI" class="Bool (strict)"() -> ("Value"=w31:bool)  [unwired: 2 in, 2 out]
      }
    }
    frame Error {
      n191 = call "Synchronize Caller Events.vi"("Module Admin"=w410) -> ("Module Admin out"=w409:refnum<class "Delacor_lib_QMH_Cloneable Module Admin.lvclass">)  [unwired: 9 in, 1 out]
      n192 = property on="Property Node" class="Mod Admin"(reference=w409) -> ("Accessors:Module ID"=w408:i32)  [unwired: 1 in, 2 out]
      n193 = call-dynamic "Delacor_lib_QMH_Release Message Queue.vi"("error in"=w416, "Message Queue"=w407) -> ("error out"=w415:errorcluster)  [unwired: 9 in]
      n194 = call "Module Name--constant.vi"("Module ID"=w408) -> ("Module Name"=w413:string)  [unwired: 10 in]
      n195 = Format Into String(format string="An error occurred during initialization. %s is no longer running.", w413) -> (resulting string=w411:string)  [unwired: 2 in, 1 out]
      n196 = call "Error Reported.vi"("Additional Information"=w411, "Error"=w415, "Module ID"=w408) -> ()  [unwired: 8 in, 1 out]
    }
  }
  n197 = Merge Errors(w17, w16) -> (w18:errorcluster)
  n198 = call "Close Module.vi"("error in"=w18, "Wait for stop?"=w2, "Module Admin in"=w4) -> ("error out"=w14:errorcluster, "External Launch"=w1:bool, "Module Admin out"=w3:refnum<class "Delacor_lib_QMH_Cloneable Module Admin.lvclass">)  [unwired: 6 in]
  n199 = Unregister For Events(event registration refnum=w9, error in=w14) -> (error out=w13:errorcluster)
  "error out" <- w13
  n200 = case "External Launch?" shown="True" w1 {
    tunnel: w13 -> [_ w417]
    frame False {
    }
    frame True {
      n201 = case shown="No Error" w417 {
        frame No Error {
          n202 = invoke class="VI" method="FP.Close"() -> ()  [unwired: 3 in, 3 out]
        }
        frame Error {
          n203 = disable-structure shown="Default" {
            frame condition #0 (active) {
              n204 = invoke class="VI" method="FP.Open"("Activate"=TRUE ("Activate?")) -> ()  [unwired: 4 in, 5 out]
            }
            frame condition #1 {
              # "Don't show panel on error if running inside a built EXE."
            }
          }
        }
      }
    }
  }
  n205 = local write "Module Admin"(w3) -> ()
